vi "AddCharacteristic.vi"(8 "error in":errorcluster, 10 "FullName":string, 11 "StepRun in":refnum<class "StepRun.lvclass">) -> (0 "error out":errorcluster, 2 "Characteristic":refnum<class "Characteristic.lvclass">, 3 "StepRun out":refnum<class "StepRun.lvclass">)   [LabVIEW 2021, in "ProligentXMLGenerator.lvlib" / "StepRun.lvclass"]
doc: "A characteristic is a generic container of information that can be attached to many elements of the model.\nEach characteristic is identified by a FullName that must be unique for its owner.\nIt stores its value in a Value element.\nCharacteristics are unique among siblings by their FullName property.\nA characteristic is uniquely identified by the combination of its owner's identifier and its FullName."
uses:
  StepRun.lvclass
  StepRun.lvclass/StepRun.ctl
  Model/Characteristic/Characteristic.lvclass
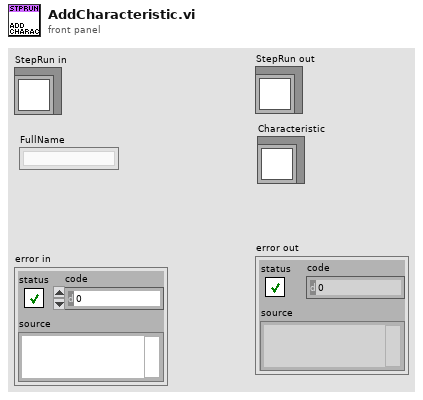
[diagram p1: front panel]
types:
  T1 = typedef "ProligentXMLGenerator.lvlib/StepRun.lvclass/Data.ctl" = cluster{"Name":string, "Measures":refnum<class "Measure.lvclass">[], "FailureReferences":refnum<class "FailureReference.lvclass">[], "Characteristics":refnum<class "Characteristic.lvclass">[], "Documents":refnum<class "Document.lvclass">[], "CustomData":refnum<class "CustomData.lvclass">, "StepExecutionStatus":refnum<class "ExecutionStatus.lvclass">, "StepRunId":refnum<class "Guid.lvclass">, "StepName":refnum<class "NonEmptyString_255.lvclass">, "StartDate":refnum<class "DateTime.lvclass">, "EndDate":refnum<class "DateTime.lvclass">, "TimeZoneInfoId":string}
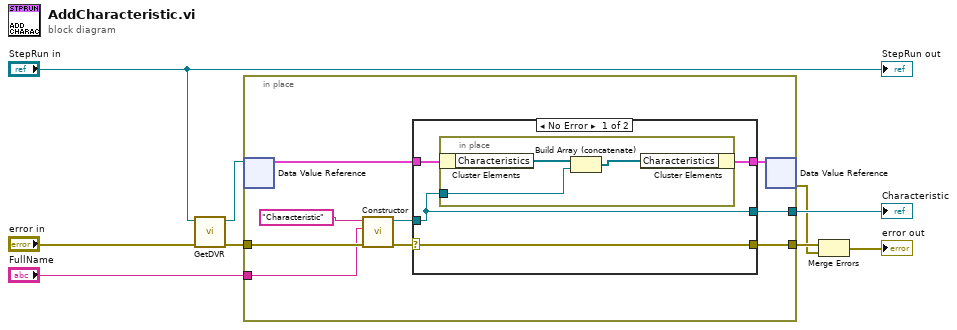
[diagram p0: block diagram]
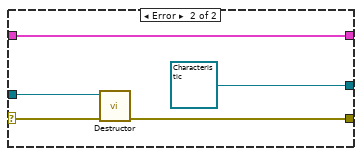
[diagram p2: hidden frame]
diagram:
  n1 = call "GetDVR.vi"("error in"="error in", "StepRun"="StepRun in") -> ("error out"=w4:errorcluster, "DVRReference"=w3:refnum<data-value>)  [unwired: 8 in]
  n2 = in-place "In Place Element Structure" {
    in-place-border: [w18] -> w5
    in-place-border: w4 -> [w11]
    in-place-border: [w15] -> w6
    in-place-border: "FullName" -> [w10]
    n3 = in-place-dvr #1(w3) -> (w17:T1)  [unwired: 1 out]
    n4 = call "Constructor.vi"("error in"=w11, "FullName"=w10, "Name"="Characteristic") -> ("error out"=w13:errorcluster, "Document out"=w14:refnum<class "Characteristic.lvclass">)  [unwired: 7 in]
    n5 = case shown="No Error" w13 {
      selector: w13 -> [w22 w29]
      tunnel: [w19 w30] -> w16
      tunnel: [w22 w28] -> w18
      tunnel: w14 -> [w21 w27]
      tunnel: w17 -> [w20 w30]
      tunnel: [w21 refnum<class "Characteristic.lvclass"> refnum ("ProligentResultProcessor:Characteristic")] -> w15
      frame No Error {
        n6 = in-place "In Place Element Structure" {
          in-place-border: w21 -> [w25]
          n7 = in-place-cluster #2(w20) -> ("Characteristics"=w24:refnum<class "Characteristic.lvclass">[])
          n8 = Build Array (concatenate)(w24, w25) -> (w23:refnum<class "Characteristic.lvclass">[])
          n9 = in-place-cluster #2("Characteristics"=w23) -> (w19:T1)
        }
      }
      frame Error {
        n10 = call "Destructor.vi"("error in"=w29, "Document in"=w27) -> ("error out"=w28:errorcluster)  [unwired: 9 in]
      }
    }
    n11 = in-place-dvr #1(w16) -> (w2:errorcluster)  [unwired: 1 out]
  }
  "Characteristic" <- w6
  n12 = Merge Errors(w5, w2) -> (→"error out":errorcluster)
  "StepRun out" <- "StepRun in"
